vi "Write Device.lvclass.vi"(10 "Device.lvclass":refnum<class "Device.lvclass">, 11 "Measurements in":refnum<class "Measurement.lvclass">) -> (3 "Measurements out":refnum<class "Measurement.lvclass">)   [LabVIEW 2020, in "Measurement.lvclass"]
uses:
  Measurement.lvclass
  Devices/Device.lvclass
  Measurement.lvclass/Measurement.ctl
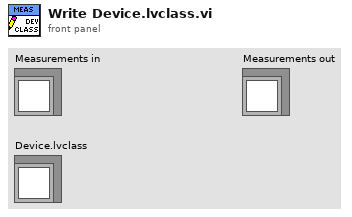
[diagram p1: front panel]
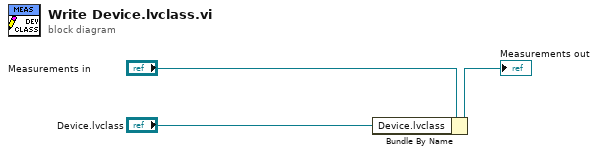
[diagram p0: block diagram]
diagram:
  n1 = Bundle By Name(cluster="Measurements in", "Device.lvclass"="Device.lvclass") -> (→"Measurements out":refnum<class "Measurement.lvclass">)
